vi "subscriber state machine.vi"(11 "subscriber":refnum<class "subscriber.lvclass">) -> ()   [LabVIEW 2015, in "subscriber.lvclass"]
uses:
  subscriber.lvclass
  communicator/communicator.lvclass/communicator.ctl
  communicator queue/identifying queue.lvclass
  communicator queue/identifying queue.lvclass/identifying queue.ctl
  message/communicator message.lvclass/communicator message.ctl
  communicator queue/enqueue variety.ctl
  message/Read data.vi
  message/set sender.vi
  communicator/communicator.lvclass
  message/communicator message.lvclass
  connection/connection maintainer.lvclass
  manager/queue manager.lvclass
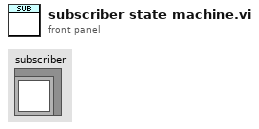
[diagram p1: front panel]
types:
  T1 = typedef "identifying queue.lvclass/enqueue variety.ctl" = enum16{"normal", "lossy", "priority"}
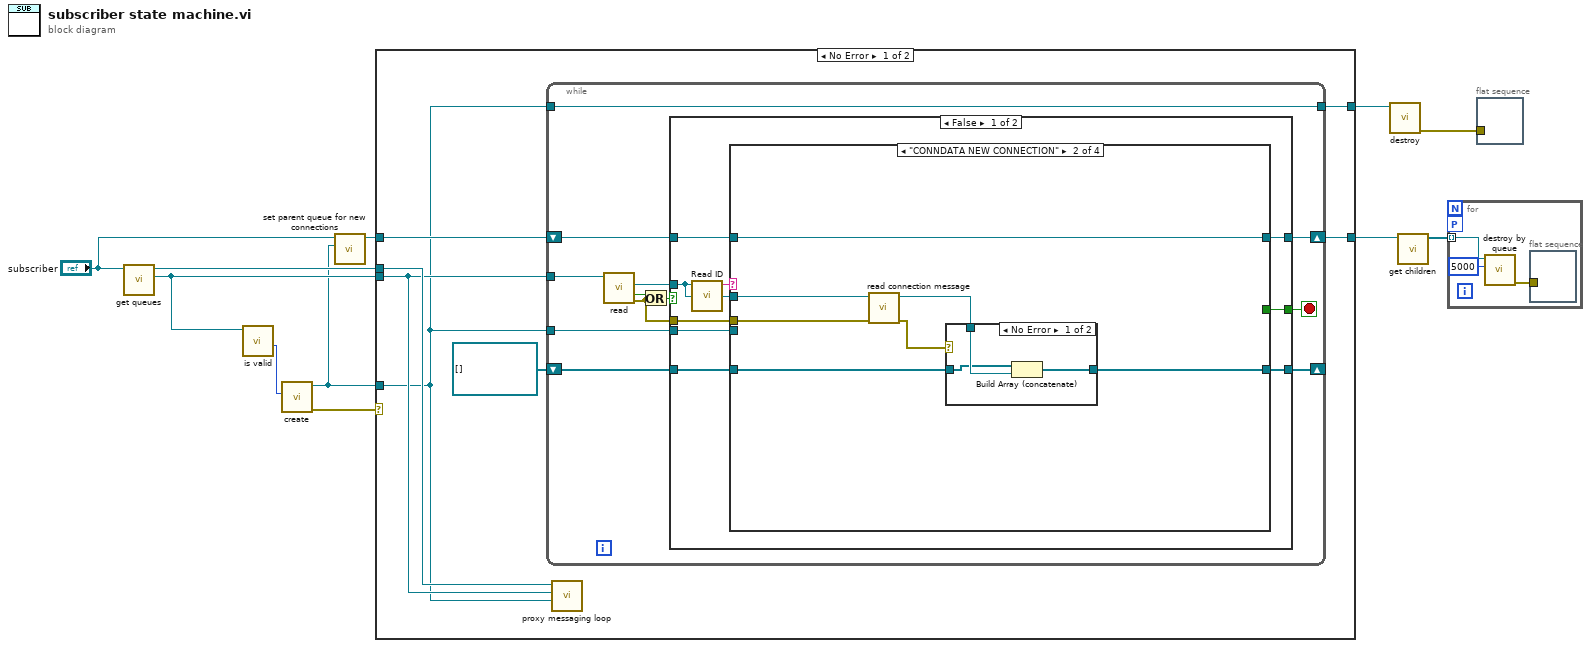
[diagram p0: block diagram]
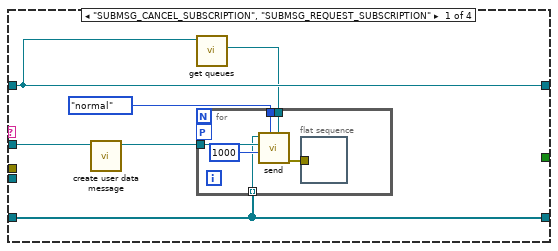
[diagram p2: hidden frame]
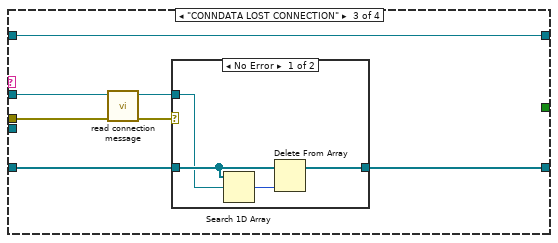
[diagram p4: hidden frame]
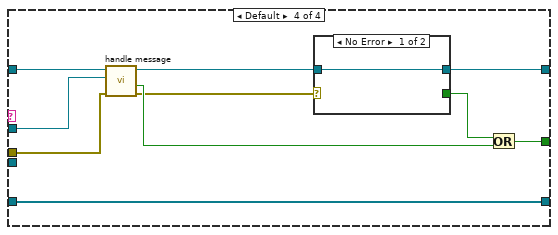
[diagram p6: hidden frame]
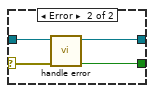
[diagram p7: hidden frame]
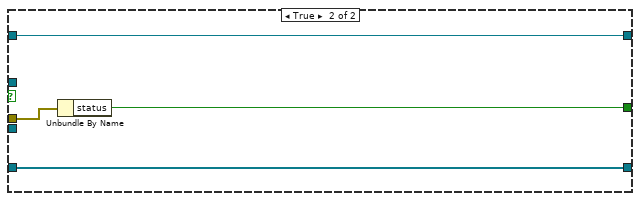
[diagram p8: hidden frame]
diagram:
  n1 = call "get queues.vi"("communicator in"="subscriber") -> ("to this"=w9:refnum<class "identifying queue.lvclass">, "to parent"=w11:refnum<class "identifying queue.lvclass">)  [unwired: 9 in]
  n2 = call "is valid.vi"("identifying queue in"=w9) -> ("max queue size"=w10:i32)  [unwired: 9 in, 1 out]
  n3 = call "create.vi"("size (1,10000)"=w10) -> ("error out"=w8:errorcluster, "message connection out"=w1:refnum<class "identifying queue.lvclass">)  [unwired: 9 in]
  n4 = call "set parent queue for new connections.vi"("conn parent queue"=w1, "queue manager in"="subscriber") -> ("queue manager out"=w2:refnum<class "subscriber.lvclass">)  [unwired: 9 in]
  n5 = case shown="No Error" w8 {
    tunnel: w9 -> [w13 _]
    tunnel: w11 -> [w14 _]
    tunnel: w1 -> [w12 w95]
    tunnel: [w17 w95] -> w7
    tunnel: w2 -> [w16 w94]
    tunnel: [w15 w94] -> w3
    frame No Error {
      n6 = while {
        tunnel: w13 -> [w24]
        shift-right: [w28] -> _
        shift-left: refnum<class "identifying queue.lvclass">[] [] -> [w27]
        tunnel: [w26] -> w17
        tunnel: w12 -> [w26]
        tunnel: w12 -> [w25]
        shift-right: [w19] -> w15
        shift-left: w16 -> [w20]
        stop <- w29 stop-if-true
        n7 = call "read.vi"("identifying queue in"=w24) -> ("error out"=w21:errorcluster, "timed out?"=w22:bool, "message"=w23:refnum<class "communicator message.lvclass">)  [unwired: 8 in]
        n8 = Or(x=w22, y=w21) -> (x .or. y?=w30:bool)
        n9 = case shown="False" w30 {
          tunnel: w21 -> [w36 w93]
          tunnel: [w38 w92] -> w29
          tunnel: w23 -> [w37 _]
          tunnel: [w35 w91] -> w28
          tunnel: w27 -> [w34 w91]
          tunnel: w25 -> [w33 _]
          tunnel: w20 -> [w32 w90]
          tunnel: [w31 w90] -> w19
          frame False {
            n10 = call "Read ID.vi"("communicator message in"=w37) -> ("ID"=w39:string)  [unwired: 10 in]
            n11 = case shown="\"CONNDATA NEW CONNECTION\"" w39 {
              tunnel: [_ _ _ w79] -> w38
              tunnel: w37 -> [w43 w58 w68 w75]
              tunnel: w36 -> [_ w57 w69 w76]
              tunnel: [w45 w55 w66 w84] -> w35
              tunnel: w34 -> [w45 w54 w65 w84]
              tunnel: w33 -> [_ _ _ _]
              tunnel: w32 -> [w42 w52 w63 w78]
              tunnel: [w42 w52 w63 w77] -> w31
              frame "SUBMSG_CANCEL_SUBSCRIPTION", "SUBMSG_REQUEST_SUBSCRIPTION" {
                n12 = call "create user data message.vi"("data"=w43) -> ("message"=w40:refnum<class "communicator message.lvclass">)  [unwired: 10 in]
                n13 = call "get queues.vi"("communicator in"=w42) -> ("to this"=w41:refnum<class "identifying queue.lvclass">)  [unwired: 9 in, 1 out]
                n14 = for {
                  workers-P: _ -> [_]
                  tunnel: w40 -> [w51]
                  tunnel: enqueue_variety."normal" ("enqueue setting") -> [w50]
                  tunnel: w45 -> [w48] mode=indexing
                  tunnel: w41 -> [w46]
                  n15 = call "send.vi"("sender"=w46, "enqueue command"=w50, "timeout in ms (-1)"=1000, "message"=w51, "message connection in"=w48) -> ("error out"=w47:errorcluster)  [unwired: 5 in, 1 out]
                  n16 = flat-sequence {
                    tunnel: w47 -> [_]
                    frame #0 {
                    }
                  }
                }
              }
              frame "CONNDATA NEW CONNECTION" {
                n17 = call "read connection message.vi"("error in"=w57, "communicator message in"=w58) -> ("error out"=w53:errorcluster, "queue"=w56:refnum<class "identifying queue.lvclass">)  [unwired: 8 in]
                n18 = case shown="No Error" w53 {
                  tunnel: w56 -> [w61 _]
                  tunnel: [w60 w62] -> w55
                  tunnel: w54 -> [w59 w62]
                  frame No Error {
                    n19 = Build Array (concatenate)(w59, w61) -> (w60:refnum<class "identifying queue.lvclass">[])
                  }
                  frame Error {
                  }
                }
              }
              frame "CONNDATA LOST CONNECTION" {
                n20 = call "read connection message.vi"("error in"=w69, "communicator message in"=w68) -> ("error out"=w67:errorcluster, "queue"=w64:refnum<class "identifying queue.lvclass">)  [unwired: 8 in]
                n21 = case shown="No Error" w67 {
                  tunnel: [w71 w74] -> w66
                  tunnel: w65 -> [w72 w74]
                  tunnel: w64 -> [w70 _]
                  frame No Error {
                    n22 = Search 1D Array(1D array=w72, element=w70) -> (index of element=w73:i32)  [unwired: 1 in]
                    n23 = Delete From Array(array=w72, index=w73) -> (array with subset deleted=w71:refnum<class "identifying queue.lvclass">[])  [unwired: 1 in, 1 out]
                  }
                  frame Error {
                  }
                }
              }
              frame Default {
                n24 = call-dynamic "handle message.vi"("error in"=w76, "message"=w75, "queue manager in"=w78) -> ("error out"=w81:errorcluster, "stop"=w82:bool, "queue manager out"=w83:refnum<class "subscriber.lvclass">)  [unwired: 6 in]
                n25 = case shown="No Error" w81 {
                  selector: w81 -> [_ w87]
                  tunnel: w83 -> [w85 w89]
                  tunnel: [w85 w88] -> w77
                  tunnel: [_ w86] -> w80
                  frame No Error {
                  }
                  frame Error {
                    n26 = call-dynamic "handle error.vi"("error in"=w87, "communicator in"=w89) -> ("unrecoverable?"=w86:bool, "communicator out"=w88:refnum<class "subscriber.lvclass">)  [unwired: 8 in]
                  }
                }
                n27 = Or(x=w80, y=w82) -> (x .or. y?=w79:bool)
              }
            }
          }
          frame True {
            n28 = Unbundle By Name(w93) -> ("status"=w92:bool)
          }
        }
      }
      n29 = call "proxy messaging loop.vi"("proxy queue"=w12, "to this"=w13, "to parent application"=w14) -> ()  [unwired: 9 in]
    }
    frame Error {
    }
  }
  n30 = call "destroy.vi"("message connection in"=w7) -> ("error out"=w6:errorcluster)  [unwired: 10 in]
  n31 = call "get children.vi"("communicator in"=w3) -> ("children"=w4:refnum<class "identifying queue.lvclass">[])  [unwired: 10 in]
  n32 = for {
    workers-P: _ -> [_]
    tunnel: w4 -> [w96] mode=indexing
    n33 = call "destroy by queue.vi"("timeout in ms (-1)"=5000, "queue"=w96) -> ("error out"=w97:errorcluster)  [unwired: 8 in, 1 out]
    n34 = flat-sequence {
      tunnel: w97 -> [_]
      frame #0 {
      }
    }
  }
  n35 = flat-sequence {
    tunnel: w6 -> [_]
    frame #0 {
    }
  }
